vi "Block DMA Benchmark.vi"() -> ()   [LabVIEW 2020]
uses:
  Source/Typedefs/GE 5565PIORC.Typedef.DMA Wait Mode.ctl
  <vilib>/Platform/TimedLoop/XDataNode/timing_clust.ctl
  <vilib>/Platform/TimedLoop/XDataNode/nitl_modes.ctl
  <vilib>/Platform/TimedLoop/XDataNode/wakeup.ctl
  Source/GE 5565PIORC.lvclass/GE 5565PIORC.ctl
  Source/Methods/GE 5565PIORC.DMA.Create Transfer (Block).vi
  Source/Properties/Registers/GE 5565PIORC.Registers.LAS1RR.PCI Address Range.Get.vi
  Source/Methods/GE 5565PIORC.PXI Interrupts.Enable.vi
  Source/Properties/Registers/GE 5565PIORC.Registers.DMACSR0.Channel 0 Enable.Set.vi
  Source/Properties/Registers/GE 5565PIORC.Registers.INTCSR.Local DMA Channel 0 Interrupt Enable.Set.vi
  Source/Methods/GE 5565PIORC.DMA.Create Transfer (Scatter-Gather).vi
  Source/Properties/Registers/GE 5565PIORC.Registers.DMADPR0.Direction of Transfer.Set.vi
  Source/Properties/Registers/GE 5565PIORC.Registers.DMASIZ0.DMA Transfer Size.Set.vi
  Source/Methods/GE 5565PIORC.DMA.Size.vi
  Source/Properties/Registers/GE 5565PIORC.Registers.DMALADR0.Local Address Register.Set.vi
  Source/Properties/Registers/GE 5565PIORC.Registers.DMAMODE0.Scatter-Gather Mode.Set.vi
  Source/Properties/Registers/GE 5565PIORC.Registers.DMAPADR0.PCI Address Register.Set.vi
  Source/Methods/GE 5565PIORC.DMA.Scatter-Gather.Link Block Descriptors.vi
  Source/Methods/GE 5565PIORC.DMA.Scatter-Gather.Commit Linked Block Descriptors.vi
  Source/Properties/Registers/GE 5565PIORC.Registers.DMADPR0.Channel 0 First Descriptor Address.Set.vi
  Source/Methods/GE 5565PIORC.DMA.Get Transfer Components.vi
  Source/Methods/GE 5565PIORC.DMA.Get Transfer Components (Scatter-Gather).vi
  Source/Properties/Registers/GE 5565PIORC.Registers.DMACSR0.Channel 0 Start.Set.vi
  Source/Properties/Registers/GE 5565PIORC.Registers.DMACSR0.Channel 0 Clear Interrupt.Set.vi
  Source/Methods/GE 5565PIORC.DMA.Poll for Done Signal.vi
  Source/Methods/GE 5565PIORC.PXI Interrupts.Wait for Event.vi
  Source/Properties/Registers/GE 5565PIORC.Registers.Local Configuration.Read.vi
  Source/Properties/Registers/GE 5565PIORC.Registers.Local Configuration.Read (U32).vi
  Source/Properties/Registers/GE 5565PIORC.Registers.Local Configuration.Read (U8).vi
  Source/Properties/Registers/GE 5565PIORC.Registers.Local Configuration.Write.vi
  Source/Properties/Registers/GE 5565PIORC.Registers.Local Configuration.Write (U8).vi
  Source/Methods/GE 5565PIORC.Bit Manipulation.Set Bit.vi
  Source/Methods/GE 5565PIORC.Bit Manipulation.Set Bit (U8).vi
  Source/Properties/Registers/GE 5565PIORC.Registers.Local Configuration.Write (U32).vi
  Source/Methods/GE 5565PIORC.Bit Manipulation.Set Bit (U32).vi
  Source/Methods/GE 5565PIORC.DMA.Scatter-Gather.Set Descriptor Params.vi
  Source/Methods/GE 5565PIORC.DMA.Is Done.vi
  <vilib>/Utility/error.llb/Clear Errors.vi
  Source/Methods/GE 5565PIORC.Registers.Read.vi
  Source/Methods/GE 5565PIORC.Registers.Read (U32).vi
  Source/Methods/GE 5565PIORC.Registers.Read (U8).vi
  Source/Methods/GE 5565PIORC.Registers.Write.vi
  Source/Methods/GE 5565PIORC.Registers.Write (U8).vi
  Source/Methods/GE 5565PIORC.Registers.Write (U32).vi
  Source/Properties/Registers/GE 5565PIORC.Registers.DMACSR0.Channel 0 Inactive.Get.vi
  Source/Methods/GE 5565PIORC.Bit Manipulation.Get Bit.vi
  Source/Methods/GE 5565PIORC.Bit Manipulation.Get Bit (U8).vi
  Source/Methods/GE 5565PIORC.Round Up to Nearest 8.vi
  Source/Methods/GE 5565PIORC.Round Up to Nearest 16.vi
  Source/GE 5565PIORC.lvclass
  <vilib>/platform/TimedLoop/XDataNode/XDataNode.xnode
  <vilib>/Platform/TimedLoop/XDataNode/XDNodeRunTimeDep.lvlib
panel:
  out "Progress":dbl(slide) scale=0.0..1.0
  in  "Increment":i32=1000
  in  "Count":i32=1000
  out "Throughput":cluster{"X":dbl, "Y":dbl}[](graph)
  in  "Transfer Direction":enum16{"Host to RFM", "RFM to Host"}(ring)=enum."RFM to Host"
  in  "Processor":i32
  in  "Wait Mode":T1=enum."Interrupt"
  in  "VISA Resource Name":refnum<visa-resource-name>="PXI4::14::INSTR"
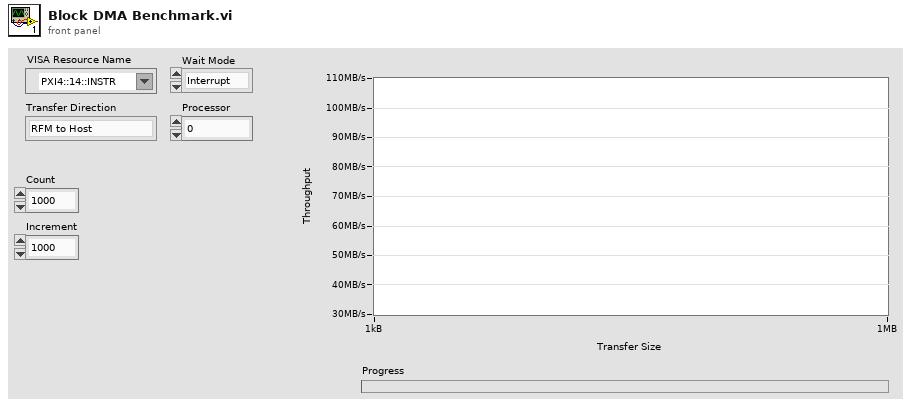
[diagram p1: front panel]
types:
  T1 = typedef "GE 5565PIORC.lvclass/GE 5565PIORC.Typedef.DMA Wait Mode.ctl" = enum16{"Polling", "Interrupt"}
  T2 = typedef "XDNodeRunTimeDep.lvlib/timing_clust.ctl" = cluster{"Expected End [f-1]":u64, "Actual End [f-1]":u64, "Finished Late? [f-1]":bool, "Expected End [i-1]":u64, "Actual End [i-1]":u64, "Finished Late? [i-1]":bool, "Expected Start [i]":u64, "Actual Start [i]":u64, "Expected Start [f]":u64, "Actual Start [f]":u64, "Source Name":string, "Structure Name":string, "Period":i64, "Deadline":i64, "Offset":i64, "Start":i64, "Priority":i32, "Timeout":i32, "Mode":T3, "Wakeup Reason":T4, "Error":errorcluster, "Source Type":string, "Secondary Source Type":string, "Global End Time":u64, "Global Start Time":u64, "Frame Duration":u64, "Iteration Duration":u64, "Assigned CPU":i32, "I/O Scan Engine Mode":u32}
  T3 = typedef "XDNodeRunTimeDep.lvlib/nitl_modes.ctl" = enum32{"No Change", "Process missed periods, maintain original phase", "Discard missed periods, maintain original phase", "Process missed periods, ignore original phase", "Discard missed periods, ignore original phase"}
  T4 = typedef "XDNodeRunTimeDep.lvlib/wakeup.ctl" = enum32{"Normal", "Aborted", "Asynchronous wakeup", "Timing source error", "Timed loop error", "Timeout"}
  T5 = typedef "GE 5565PIORC.lvclass/GE 5565PIORC.Typedef.DMA Block Descriptor.ctl" = cluster{"descriptor ptr (VISA)":u32, "descriptor ptr (RFM)":u32, "descriptor size":u32, "descriptor params":T6}
  T6 = typedef "GE 5565PIORC.lvclass/GE 5565PIORC.Typedef.DMA Block Descriptor Params.ctl" = cluster{"data ptr (lower)":u32, "data ptr (upper)":u32, "data size":u32, "next descriptor ptr":u32}
  T7 = typedef "GE 5565PIORC.lvclass/GE 5565PIORC.Typedef.DMA Transfer Spec.ctl" = cluster{"RFM offset":u32, "Block Descriptors":T5[]}
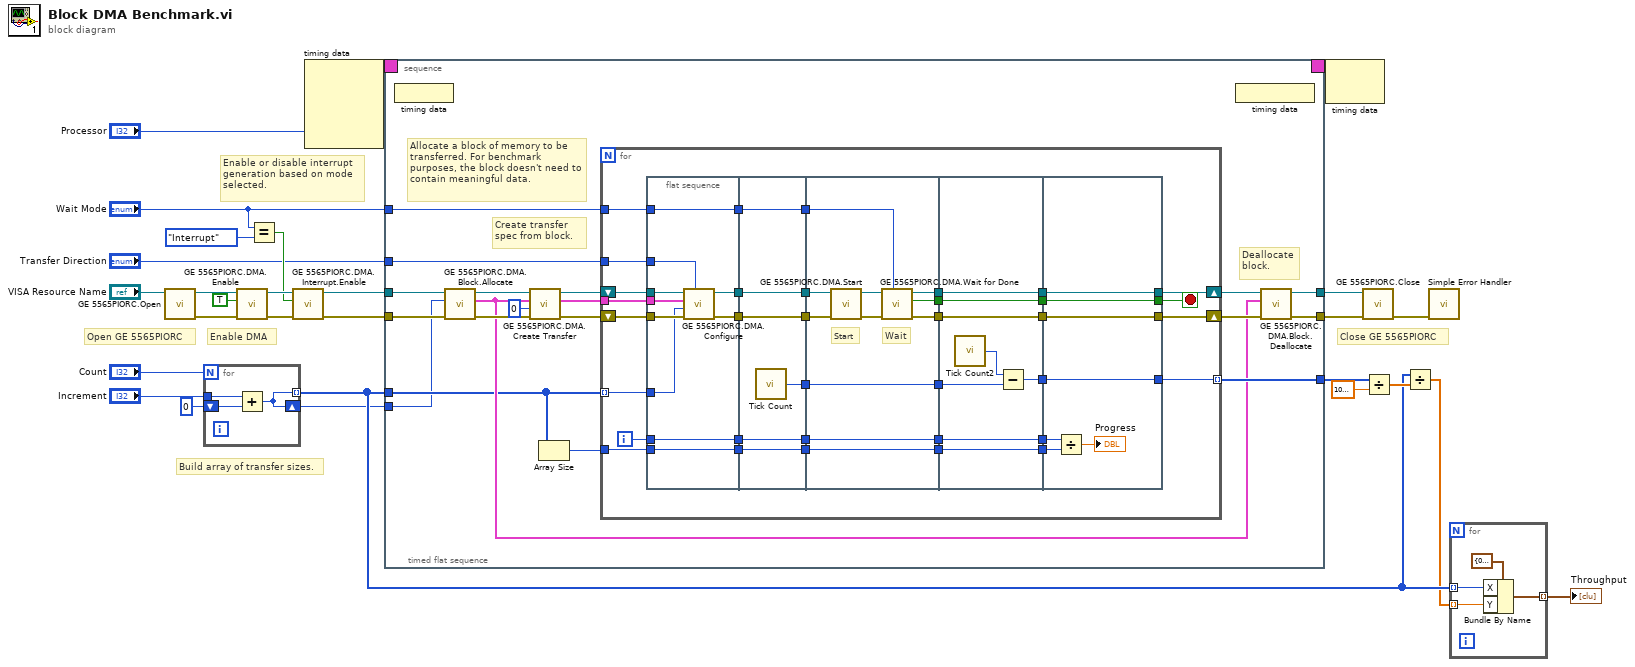
[diagram p0: block diagram]
diagram:
  # "Build array of transfer sizes."
  # "Close GE 5565PIORC"
  # "Enable or disable interrupt generation based on mode selected."
  # "Enable DMA"
  # "Open GE 5565PIORC"
  n1 = call "GE 5565PIORC.Open.vi"("VISA resource name"="VISA Resource Name") -> ("error out"=w27:errorcluster, "GE 5565PIORC"=w28:refnum<class "GE 5565PIORC.lvclass">)  [unwired: 9 in]
  n2 = for {
    N: "Count" -> [_]
    shift-right: [w31] -> w3
    shift-left: 0 -> [w29]
    tunnel: [w31] -> w6 mode=indexing
    tunnel: "Increment" -> [w30]
    n3 = Add(x=w30, y=w29) -> (x+y=w31:i32)
  }
  n4 = call "GE 5565PIORC.DMA.Enable.vi"("error in (no error)"=w27, "enable (T)"=TRUE, "GE 5565PIORC in"=w28) -> ("error out"=w25:errorcluster, "GE 5565PIORC out"=w24:refnum<class "GE 5565PIORC.lvclass">)  [unwired: 7 in]
  n5 = Equal?(x="Wait Mode", y=GE_5565PIORC.Typedef.DMA_Wait_Mode."Interrupt") -> (x = y?=w22:bool)
  n6 = call "GE 5565PIORC.DMA.Interrupt.Enable.vi"("error in (no error)"=w25, "enable (T)"=w22, "GE 5565PIORC in"=w24) -> ("error out"=w12:errorcluster, "GE 5565PIORC out"=w13:refnum<class "GE 5565PIORC.lvclass">)  [unwired: 7 in]
  n7 = node-c288("Processor") -> (w18:T2)  [unwired: 3 in]
  n8 = timed-sequence {
    timing: w18 -> [_]
    timing-out: [_] -> w17
    tunnel: w13 -> [w38]
    tunnel: w12 -> [w37]
    tunnel: "Wait Mode" -> [w36]
    tunnel: [w40] -> w20
    tunnel: [w39] -> w8
    tunnel: [w35] -> w9
    tunnel: w6 -> [w33]
    tunnel: w3 -> [w34]
    tunnel: "Transfer Direction" -> [w32]
    n9 = timed-flat-sequence {
      tunnel: [w59] -> w40
      tunnel: [w58] -> w39
      tunnel: w37 -> [w56]
      tunnel: w38 -> [w57]
      tunnel: w36 -> [w55]
      tunnel: [w54] -> w35
      tunnel: w34 -> [w41]
      tunnel: w33 -> [w43]
      tunnel: w32 -> [w47]
      # "Deallocate block."
      # "Create transfer spec from block."
      # "Allocate a block of memory to be transferred. For benchmark purposes, the block doesn't need to contain meaningful data."
      n10 = node-c288() -> ()  [unwired: 1 in]
      n11 = call "GE 5565PIORC.DMA.Block.Allocate.vi"("error in (no error)"=w56, "size in bytes"=w41, "GE 5565PIORC in"=w57) -> ("error out"=w46:errorcluster, "Block Descriptor"=w44:T5, "GE 5565PIORC out"=w45:refnum<class "GE 5565PIORC.lvclass">)  [unwired: 6 in]
      n12 = call-poly "GE 5565PIORC.DMA.Create Transfer.vi"("error in (no error)"=w46, "RFM offset"=u32 0, "Block Descriptor"=w44, "GE 5565PIORC in"=w45) -> ("error out"=w50:errorcluster, "DMA Transfer Spec"=w49:T7, "GE 5565PIORC out"=w51:refnum<class "GE 5565PIORC.lvclass">)  [unwired: 4 in, 1 out]
      n13 = Array Size(array=w43) -> (size(s)=w42:i32)
      n14 = for {
        shift-right: [w86] -> w53
        shift-left: w51 -> [w96]
        shift-right: [w85] -> w52
        shift-left: w50 -> [w95]
        tunnel: w55 -> [w91]
        tunnel: [w84] -> w54 mode=indexing
        tunnel: w49 -> [w78]
        tunnel: w43 -> [w77] mode=indexing
        tunnel: w47 -> [w76]
        tunnel: w42 -> [w70]
        i -> [w71]
        stop <- w82 stop-if-true
        n15 = flat-sequence {
          tunnel: w91 -> [w106]
          tunnel: w95 -> [w104]
          tunnel: w96 -> [w105]
          tunnel: [w106] -> w81
          tunnel: [w103] -> w80
          tunnel: [w102] -> w79
          tunnel: w78 -> [w101]
          tunnel: w77 -> [w100]
          tunnel: w76 -> [w99]
          tunnel: w71 -> [w98]
          tunnel: w70 -> [w97]
          tunnel: [w98] -> w66
          tunnel: [w97] -> w62
          tunnel: [w112] -> w94
          tunnel: [w111] -> w93
          tunnel: [w110] -> w92
          tunnel: [w109] -> w90
          tunnel: w81 -> [w109]
          tunnel: w80 -> [w111]
          tunnel: w79 -> [w110]
          tunnel: [w108] -> w67
          tunnel: w66 -> [w108]
          tunnel: [w107] -> w63
          tunnel: w62 -> [w107]
          tunnel: w94 -> [w123]
          tunnel: w93 -> [w122]
          tunnel: w92 -> [w121]
          tunnel: w90 -> [w116]
          tunnel: [w123] -> w89
          tunnel: [w118] -> w88
          tunnel: [w117] -> w87
          tunnel: [w115] -> w83
          tunnel: [w114] -> w68
          tunnel: w67 -> [w114]
          tunnel: [w113] -> w64
          tunnel: w63 -> [w113]
          tunnel: w89 -> [w128]
          tunnel: w88 -> [w131]
          tunnel: w87 -> [w130]
          tunnel: w83 -> [w126]
          tunnel: [w131] -> w75
          tunnel: [w130] -> w74
          tunnel: [w127] -> w73
          tunnel: [w126] -> w72
          tunnel: [w125] -> w69
          tunnel: w68 -> [w125]
          tunnel: [w124] -> w65
          tunnel: w64 -> [w124]
          tunnel: [w135] -> w82
          tunnel: [w136] -> w84
          tunnel: [w137] -> w85
          tunnel: [w138] -> w86
          tunnel: w75 -> [w138]
          tunnel: w74 -> [w137]
          tunnel: w73 -> [w136]
          tunnel: w72 -> [w135]
          tunnel: w69 -> [w134]
          tunnel: w65 -> [w133]
          frame #0 {
            n16 = call "GE 5565PIORC.DMA.Configure.vi"("transfer direction"=w99, "error in (no error)"=w104, "transfer size (-1: all)"=w100, "DMA Transfer Spec"=w101, "GE 5565PIORC in"=w105) -> ("error out"=w102:errorcluster, "GE 5565PIORC out"=w103:refnum<class "GE 5565PIORC.lvclass">)  [unwired: 5 in]
          }
          frame #1 {
            n17 = call "Tick Count"() -> ("Tick Count(uSec)"=w112:u32)
          }
          frame #2 {
            # "Wait"
            # "Start"
            n18 = call "GE 5565PIORC.DMA.Start.vi"("error in (no error)"=w121, "GE 5565PIORC in"=w122) -> ("error out"=w119:errorcluster, "GE 5565PIORC out"=w120:refnum<class "GE 5565PIORC.lvclass">)  [unwired: 8 in]
            n19 = call "GE 5565PIORC.DMA.Wait for Done.vi"("wait mode (polling)"=w116, "error in (no error)"=w119, "GE 5565PIORC in"=w120) -> ("error out"=w117:errorcluster, "timed out?"=w115:bool, "GE 5565PIORC out"=w118:refnum<class "GE 5565PIORC.lvclass">)  [unwired: 6 in]
          }
          frame #3 {
            n20 = call "Tick Count2"() -> ("Tick Count(uSec)"=w129:u32)
            n21 = Subtract(x=w129, y=w128) -> (x-y=w127:u32)
          }
          frame #4 {
            n22 = Divide(x=w134, y=w133) -> (x/y=→"Progress":dbl)
          }
        }
      }
      n23 = node-c288() -> ()  [unwired: 1 out]
      n24 = call "GE 5565PIORC.DMA.Block.Deallocate.vi"("error in (no error)"=w52, "Block Descriptor"=w44, "GE 5565PIORC in"=w53) -> ("error out"=w58:errorcluster, "GE 5565PIORC out"=w59:refnum<class "GE 5565PIORC.lvclass">)  [unwired: 7 in]
    }
  }
  n25 = node-c288(w17) -> ()  [unwired: 1 out]
  n26 = call "GE 5565PIORC.Close.vi"("error in (no error)"=w8, "GE 5565PIORC in"=w20) -> ("error out"=w19:errorcluster)  [unwired: 8 in, 1 out]
  n27 = Divide(x=w9, y=1000000.0) -> (x/y=w14:dbl[])
  n28 = Divide(x=w6, y=w14) -> (x/y=w5:dbl[])
  n29 = call <vilib>:"Simple Error Handler.vi"("error in (no error)"=w19) -> ()  [unwired: 4 in, 5 out]
  n30 = for {
    tunnel: w6 -> [w141] mode=indexing
    tunnel: w5 -> [w140] mode=indexing
    tunnel: [w139] -> w4 mode=indexing
    n31 = Bundle By Name(cluster=cluster{"X":dbl, "Y":dbl} {"X"=0.0, "Y"=0.0}, "X"=w141, "Y"=w140) -> (w139:cluster{"X":dbl, "Y":dbl})
  }
  "Throughput" <- w4
